vi "Set and Get ItemNames With Sysmbol.vi"(7 "Mode":T3, 8 "错误输入":errorcluster, 11 "Mlistbox Ref":refnum<vi>) -> (0 "错误输出":errorcluster, 3 "Mlistbox Ref Dup":refnum<vi>)   [LabVIEW 2012, in "Mlistbox Tools.lvlib"]
uses:
  Mlistbox Tools.lvlib
  ListBox/Custom Type/Read and Write Mode.ctl
  Custom Type/ItemName With Symbol.ctl
  ListBox/Custom Type/System Symbols.ctl
  ListBox/Listbox Tool.lvlib
panel:
  out "ItemNames Out":T1[](array[typedef])
  in  "ItemNames In":T1[](array[typedef])
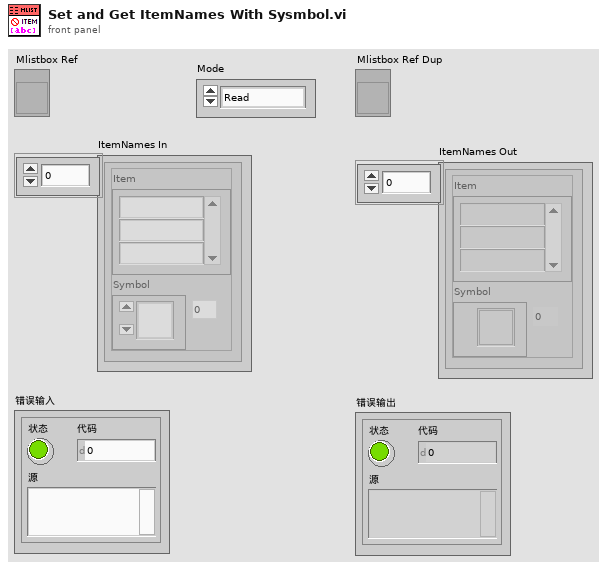
[diagram p1: front panel]
types:
  T1 = typedef "Mlistbox Tools.lvlib/ItemName With Symbol.ctl" = cluster{"Item":string[], "Symbol":T2}
  T2 = typedef "Listbox Tool.lvlib/System Symbols.ctl" = i32
  T3 = typedef "Listbox Tool.lvlib/Read and Write Mode.ctl" = enum16{"Read", "Write"}
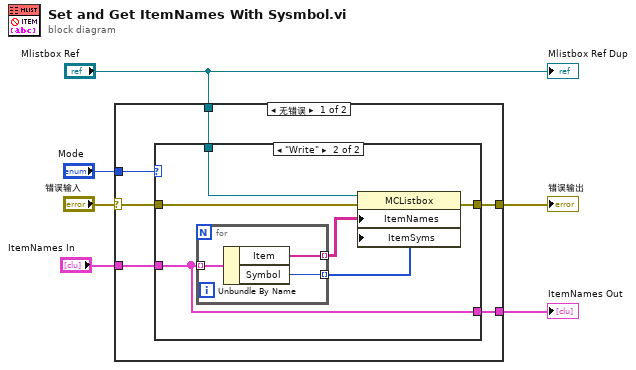
[diagram p0: block diagram]
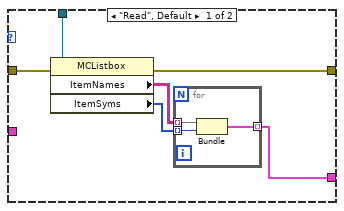
[diagram p2: hidden frame]
diagram:
  n1 = case shown="无错误" "错误输入" {
    selector: "错误输入" -> [w11 w31]
    tunnel: [w10 w31] -> w5
    tunnel: "Mode" -> [w12 _]
    tunnel: "ItemNames In" -> [w9 _]
    tunnel: [w8 _] -> w2
    tunnel: "Mlistbox Ref" -> [w7 _]
    frame No Error {
      n2 = case shown="\"Write\"" w12 {
        tunnel: w11 -> [w18 w27]
        tunnel: [w17 w26] -> w10
        tunnel: w9 -> [_ w25]
        tunnel: [w14 w25] -> w8
        tunnel: w7 -> [w13 w22]
        frame "Read", Default {
          n3 = property class="MCListbox"(reference=w13, error in=w18) -> (error out=w17:errorcluster, "ItemNames"=w16:string[][], "ItemSyms"=w15:i32[])  [unwired: 1 out]
          n4 = for {
            tunnel: w16 -> [w21] mode=indexing
            tunnel: w15 -> [w20] mode=indexing
            tunnel: [w19] -> w14 mode=indexing
            n5 = Bundle("ItemNames"=w21, w20) -> (w19:cluster{"ItemNames":string[], i32})  [unwired: 1 in]
          }
        }
        frame "Write" {
          n6 = for {
            tunnel: [w30] -> w24 mode=indexing
            tunnel: [w29] -> w23 mode=indexing
            tunnel: w25 -> [w28] mode=indexing
            n7 = Unbundle By Name(w28) -> ("Item"=w30:string[], "Symbol"=w29:T2)
          }
          n8 = property class="MCListbox"(reference=w22, error in=w27, "ItemNames"=w24, "ItemSyms"=w23) -> (error out=w26:errorcluster)  [unwired: 1 out]
        }
      }
    }
    frame Error {
    }
  }
  "错误输出" <- w5
  "ItemNames Out" <- w2
  "Mlistbox Ref Dup" <- "Mlistbox Ref"
